vi "Interface1.vi"() -> ()   [LabVIEW 2010]
panel:
  in  "stop":bool
  in  "action":bool
  out "numeric":dbl
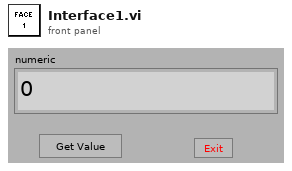
[diagram p1: front panel]
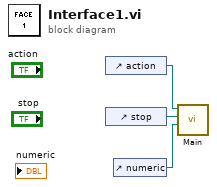
[diagram p0: block diagram]
diagram:
  n1 = control-ref of="action"() -> (w3:refnum<vi>)
  n2 = control-ref of="stop"() -> (w2:refnum<vi>)
  n3 = control-ref of="numeric"() -> (w1:refnum<vi>)
  n4 = call "Main.vi"("numeric"=w1, "stop"=w2, "get value"=w3) -> ()  [unwired: 9 in]
